vi "Set Exp to test_MultiTest.vi"(0 "Test Information":T5={"Exp Name"="Cold Switching", "Lot"="0233A", "Wafer"="15", "Die Type"="L22", "Die X "="6", "Die Y"="8", "Exp"="1", "Die X_Y"="8"}, 2 "ListBox_Selected_Tests":T1, 5 "Experiments":T4={"Exp 1"={"Floor_Sweep_Stop_V"=36.0, "Resistance Threshold"=1.0, "Floor_Sweep_Start_V"=36.0, "Floor_Sweep_Step_V"=1.0, "Roof_Sweep_Stop_V"=36.0, "Roof_Sweep_Start_V"=36.0, "Roof_Sweep_Step_V"=1.0, "Experiment Name"="", "Meas_Type"=[0, 2, 4]}, "Exp 2"={"Floor_Sweep_Stop_V"=36.0, "Resistance Threshold"=1.0, "Floor_Sweep_Start_V"=36.0, "Floor_Sweep_Step_V"=1.0, "Roof_Sweep_Stop_V"=36.0, "Roof_Sweep_Start_V"=36.0, "Roof_Sweep_Step_V"=1.0, "Experiment Name"="", "Meas_Type"=[0, 2, 4]}, "Exp 3"={"Floor_Sweep_Stop_V"=36.0, "Resistance Threshold"=1.0, "Floor_Sweep_Start_V"=36.0, "Floor_Sweep_Step_V"=1.0, "Roof_Sweep_Stop_V"=36.0, "Roof_Sweep_Start_V"=36.0, "Roof_Sweep_Step_V"=1.0, "Experiment Name"="", "Meas_Type"=[0, 2, 4]}, "Exp 4"={"Floor_Sweep_Stop_V"=36.0, "Resistance Threshold"=1.0, "Floor_Sweep_Start_V"=36.0, "Floor_Sweep_Step_V"=1.0, "Roof_Sweep_Stop_V"=36.0, "Roof_Sweep_Start_V"=36.0, "Roof_Sweep_Step_V"=1.0, "Experiment Name"="", "Meas_Type"=[0, 2, 4]}}, 11 "Error In":errorcluster) -> (4 "Selected Exp Settings":T2={"Floor_Sweep_Stop_V"=36.0, "Resistance Threshold"=1.0, "Floor_Sweep_Start_V"=36.0, "Floor_Sweep_Step_V"=1.0, "Roof_Sweep_Stop_V"=36.0, "Roof_Sweep_Start_V"=36.0, "Roof_Sweep_Step_V"=1.0, "Experiment Name"="", "Meas_Type"=[0, 2, 4]}, 6 "Test Information Out":T5={"Exp Name"="Cold Switching", "Lot"="0233A", "Wafer"="15", "Die Type"="L22", "Die X "="6", "Die Y"="8", "Exp"="1", "Die X_Y"="8"}, 8 "Per Exp Tests to Run":string[](array[string]), 15 "Error Out":errorcluster)   [LabVIEW 2013]
uses:
  Controls/Test Information.ctl
  Controls/Multiple Exp Setup_MultiTest.ctl
  Controls/Individual User Inputs_MultiTest.ctl
  Controls/Test Selection.ctl
panel:
  # "Calculation Settings"
  # "Test Settings"
  # "Calculation Settings"
  # "Test Settings"
  # "Calculation Settings"
  # "Test Settings"
  # "Calculation Settings"
  # "Test Settings"
  # "Calculation Settings"
  # "Test Settings"
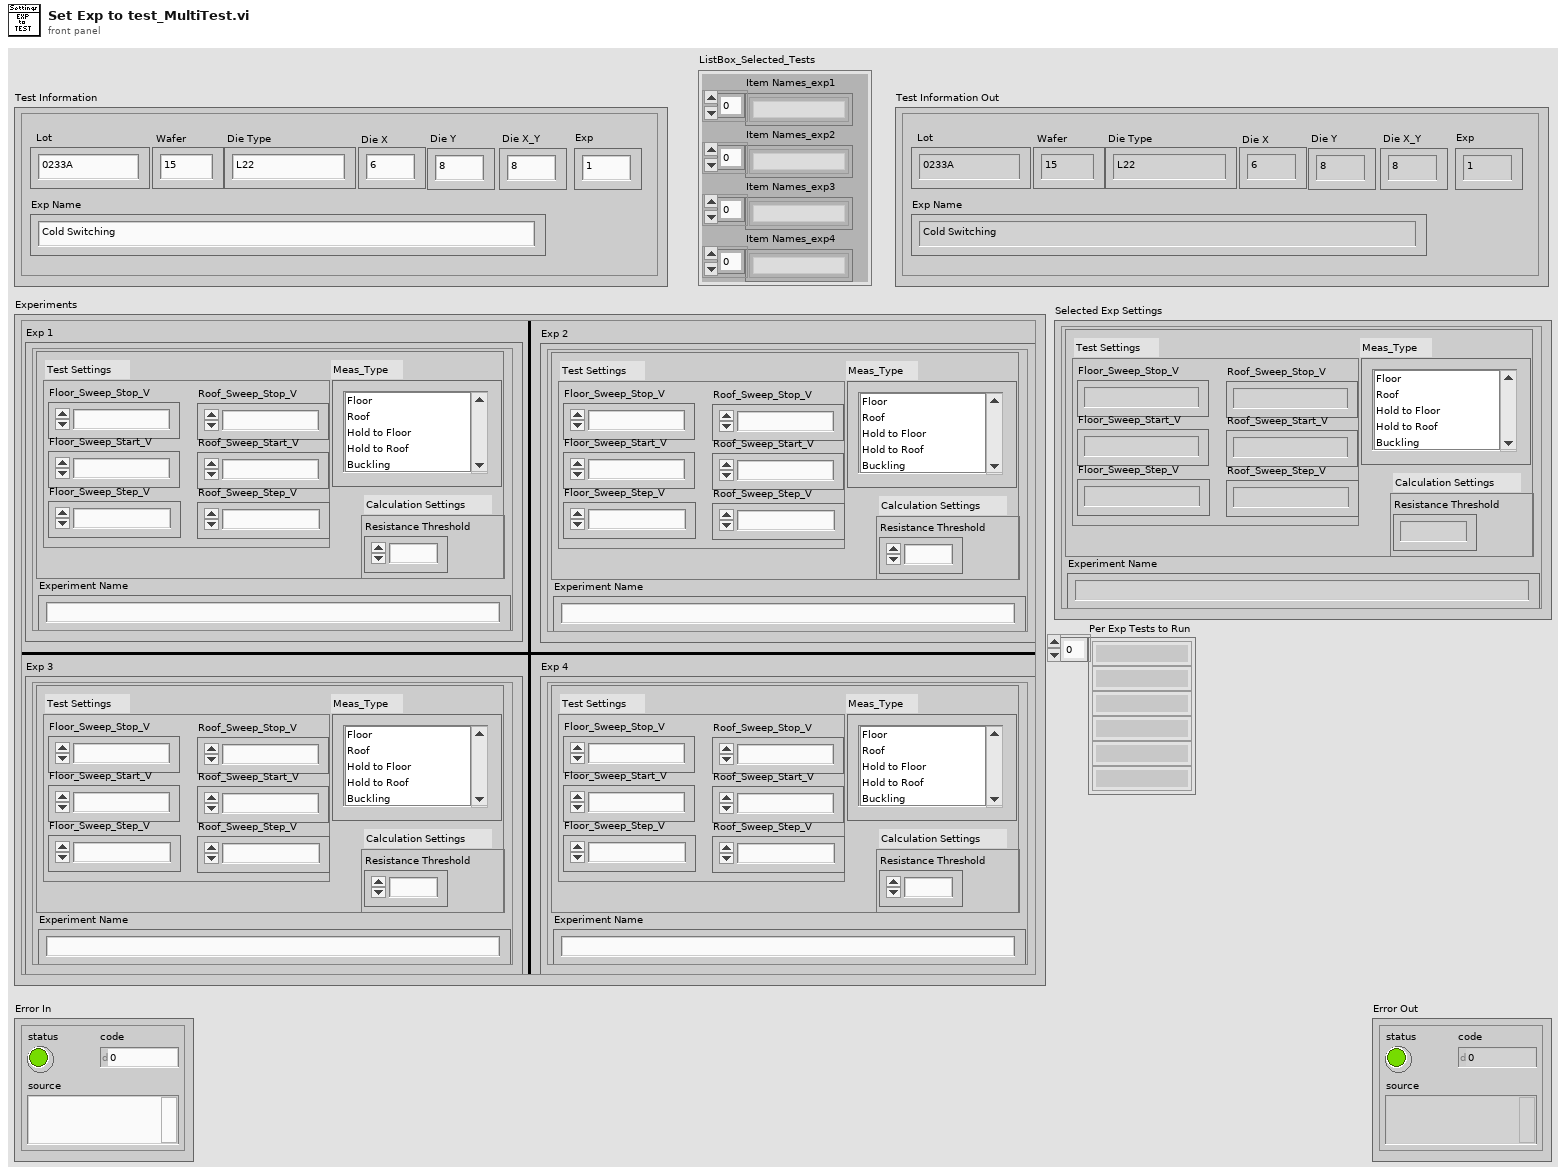
[diagram p1: front panel]
types:
  T1 = cluster{"Item Names_exp1":string[], "Item Names_exp2":string[], "Item Names_exp3":string[], "Item Names_exp4":string[]}
  T2 = typedef "Individual User Inputs_MultiTest.ctl" = cluster{"Floor_Sweep_Stop_V":dbl, "Resistance Threshold":dbl, "Floor_Sweep_Start_V":dbl, "Floor_Sweep_Step_V":dbl, "Roof_Sweep_Stop_V":dbl, "Roof_Sweep_Start_V":dbl, "Roof_Sweep_Step_V":dbl, "Experiment Name":string, "Meas_Type":T3}
  T3 = typedef "Test Selection.ctl" = i32[]
  T4 = typedef "Multiple Exp Setup_MultiTest.ctl" = cluster{"Exp 1":T2, "Exp 2":T2, "Exp 3":T2, "Exp 4":T2}
  T5 = typedef "Test Information.ctl" = cluster{"Exp Name":string, "Lot":string, "Wafer":string, "Die Type":string, "Die X ":string, "Die Y":string, "Exp":string, "Die X_Y":string}
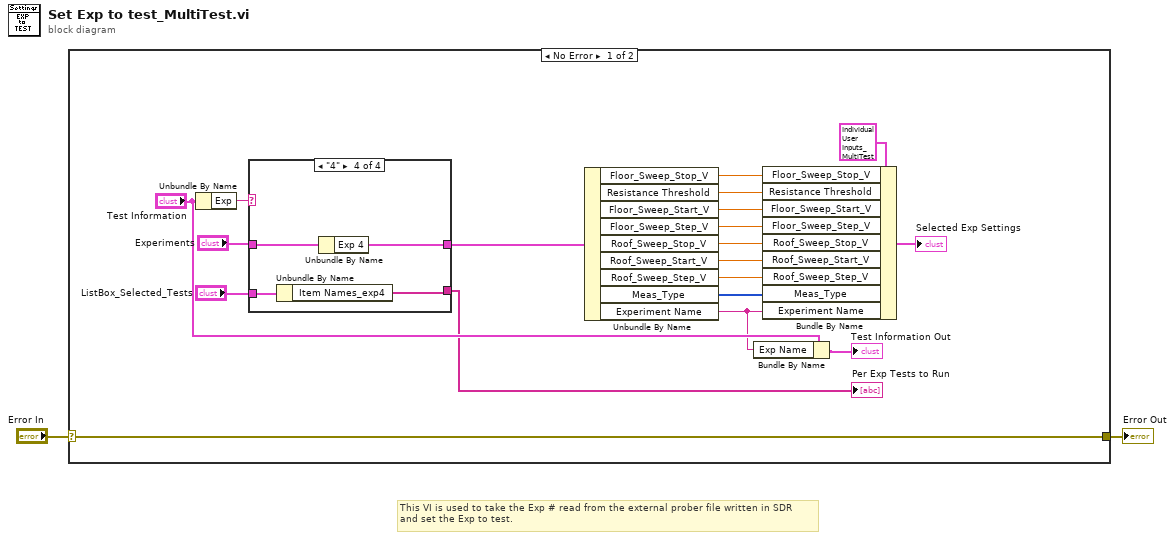
[diagram p0: block diagram]
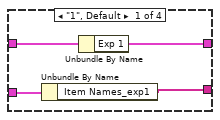
[diagram p2: hidden frame]
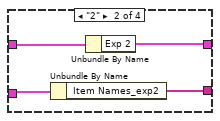
[diagram p3: hidden frame]
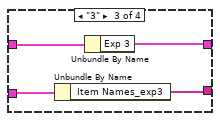
[diagram p4: hidden frame]
diagram:
  # "This VI is used to take the Exp # read from the external prober file written in SDR\nand set the Exp to test."
  n1 = case shown="No Error" "Error In" {
    selector: "Error In" -> [w4 w38]
    tunnel: [w4 w38] -> w1
    frame No Error {
      n2 = Unbundle By Name("Test Information") -> ("Exp"=w21:string)
      n3 = case shown="\"4\"" w21 {
        tunnel: [w24 w29 w33 w37] -> w18
        tunnel: "Experiments" -> [w25 w28 w32 w36]
        tunnel: "ListBox_Selected_Tests" -> [w23 w27 w31 w35]
        tunnel: [w22 w26 w30 w34] -> w3
        frame "1", Default {
          n4 = Unbundle By Name(w23) -> ("Item Names_exp1"=w22:string[])
          n5 = Unbundle By Name(w25) -> ("Exp 1"=w24:T2)
        }
        frame "2" {
          n6 = Unbundle By Name(w27) -> ("Item Names_exp2"=w26:string[])
          n7 = Unbundle By Name(w28) -> ("Exp 2"=w29:T2)
        }
        frame "3" {
          n8 = Unbundle By Name(w31) -> ("Item Names_exp3"=w30:string[])
          n9 = Unbundle By Name(w32) -> ("Exp 3"=w33:T2)
        }
        frame "4" {
          n10 = Unbundle By Name(w35) -> ("Item Names_exp4"=w34:string[])
          n11 = Unbundle By Name(w36) -> ("Exp 4"=w37:T2)
        }
      }
      "Per Exp Tests to Run" <- w3
      n12 = Unbundle By Name(w18) -> ("Floor_Sweep_Stop_V"=w17:dbl, "Resistance Threshold"=w16:dbl, "Floor_Sweep_Start_V"=w15:dbl, "Floor_Sweep_Step_V"=w14:dbl, "Roof_Sweep_Stop_V"=w13:dbl, "Roof_Sweep_Start_V"=w12:dbl, "Roof_Sweep_Step_V"=w11:dbl, "Meas_Type"=w6:T3, "Experiment Name"=w10:string)
      n13 = Bundle By Name(cluster="Test Information", "Exp Name"=w10) -> (→"Test Information Out":T5)
      n14 = Bundle By Name(cluster=T2 {"Floor_Sweep_Stop_V"=36.0, "Resistance Threshold"=1.0, "Floor_Sweep_Start_V"=36.0, "Floor_Sweep_Step_V"=1.0, "Roof_Sweep_Stop_V"=36.0, "Roof_Sweep_Start_V"=36.0, "Roof_Sweep_Step_V"=1.0, "Experiment Name"="", "Meas_Type"=[0, 2, 4]} ("Selected Exp Settings"), "Floor_Sweep_Stop_V"=w17, "Resistance Threshold"=w16, "Floor_Sweep_Start_V"=w15, "Floor_Sweep_Step_V"=w14, "Roof_Sweep_Stop_V"=w13, "Roof_Sweep_Start_V"=w12, "Roof_Sweep_Step_V"=w11, "Meas_Type"=w6, "Experiment Name"=w10) -> (→"Selected Exp Settings":T2)
    }
    frame Error {
    }
  }
  "Error Out" <- w1
